vi "WriteVerify Mfg Test Timestamp.vi"(8 "error in":errorcluster) -> (0 "error out":errorcluster)   [LabVIEW 2015]
panel:
  out "Time Stamp":timestamp
  out "Delta Time":dbl
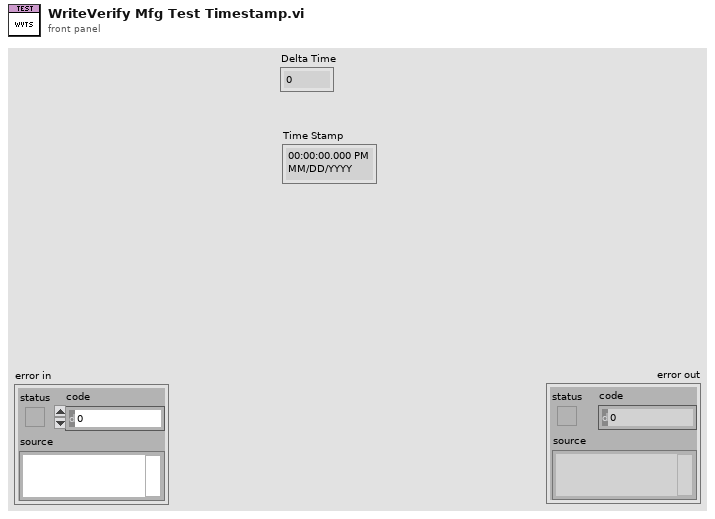
[diagram p1: front panel]
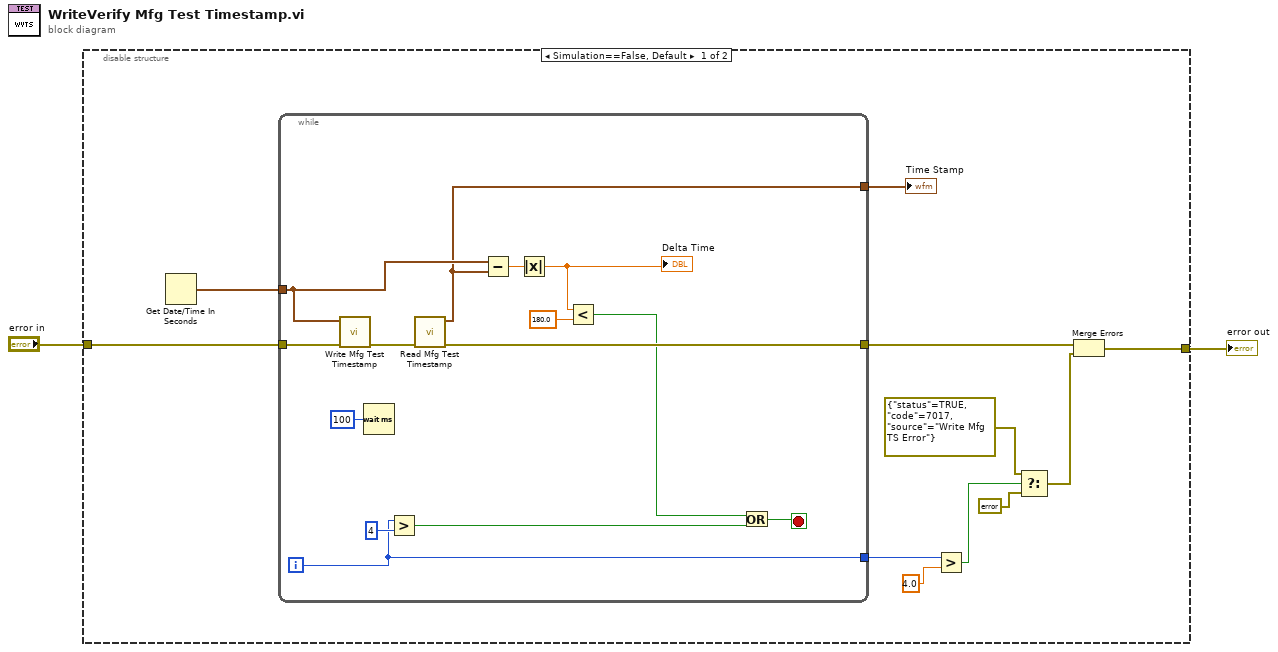
[diagram p0: block diagram]
diagram:
  n1 = disable-structure shown="Simulation==False, Default" {
    disable-tunnel: "error in" -> [w13 w28]
    disable-tunnel: [w5 w28] -> w1
    frame condition #0 (active) {
      n2 = Get Date/Time In Seconds() -> (seconds since 1Jan1904=w4:timestamp)
      n3 = while {
        tunnel: w13 -> [w27]
        tunnel: [w17] -> w6
        tunnel: [w22] -> w11
        tunnel: w4 -> [w15]
        tunnel: [w14] -> w3
        i -> [w22]
        stop <- w24 stop-if-true
        n4 = call "Write Mfg Test Timestamp.vi"("error in"=w27, "Time Stamp"=w15) -> ("error out"=w21:errorcluster)  [unwired: 9 in]
        n5 = Wait (ms)(milliseconds to wait=u32 100) -> ()  [unwired: 1 out]
        n6 = Greater?(x=w22, y=4) -> (0:w25:bool)
        n7 = call "Read Mfg Test Timestamp.vi"("error in"=w21) -> ("time stamp"=w14:timestamp, "error out"=w17:errorcluster)  [unwired: 8 in]
        n8 = Subtract(x=w15, y=w14) -> (x-y=w20:dbl)
        n9 = Absolute Value(x=w20) -> (abs(x)=w19:dbl)
        "Delta Time" <- w19
        n10 = Less?(x=w19, y=180.0) -> (x < y?=w16:bool)
        n11 = Or(x=w16, y=w25) -> (x .or. y?=w24:bool)
      }
      "Time Stamp" <- w3
      n12 = Greater?(x=w11, y=4.0) -> (0:w10:bool)
      n13 = Select(t=errorcluster {"status"=TRUE, "code"=7017, "source"="Write Mfg TS Error"} ("f"), s=w10, f=errorcluster {"status"=FALSE, "code"=0, "source"=""}) -> (s? t:f=w7:errorcluster)
      n14 = Merge Errors(w6, w7) -> (w5:errorcluster)
    }
    frame condition #1 {
    }
  }
  "error out" <- w1
